vi "PeriodicTaskChannels.vi"(7 "Error In":errorcluster, 8 "Display Type":enum8{"Matrix", "7 Segment"}(ring), 9 "Channels":T1, 10 "LINX Resource":T2) -> (0 "Error Out":errorcluster, 2 "Response":u8[](array[numeric]), 3 "LINX Resource":T2)   [LabVIEW 2019, in "LMH-LINX.lvlib" / "Interaction Parts Kit.lvlib"]
doc: "Updates the Channels used in the Periodic Task using a Custom Command"
uses:
  <vilib>/MakerHub/LINX/Public/Sensors/Digilent/Interaction Parts Kit/Interaction Parts Kit.lvlib
  <vilib>/MakerHub/LINX/Private/Type Defs/LINX Ref.ctl
  <vilib>/MakerHub/LINX/Private/Type Defs/Platform.ctl
  <vilib>/MakerHub/LINX/Private/Type Defs/Interface.ctl
  <vilib>/MakerHub/LINX/Private/Device/Type Defs/LINX Device Config.ctl
  <vilib>/MakerHub/LINX/Private/Device/Type Defs/TCP Config.ctl
  <vilib>/MakerHub/LINX/Private/Device/Type Defs/Channels.ctl
  <vilib>/MakerHub/LINX/LMH-LINX.lvlib
  <vilib>/MakerHub/LINX/Private/Device/Device.lvlib
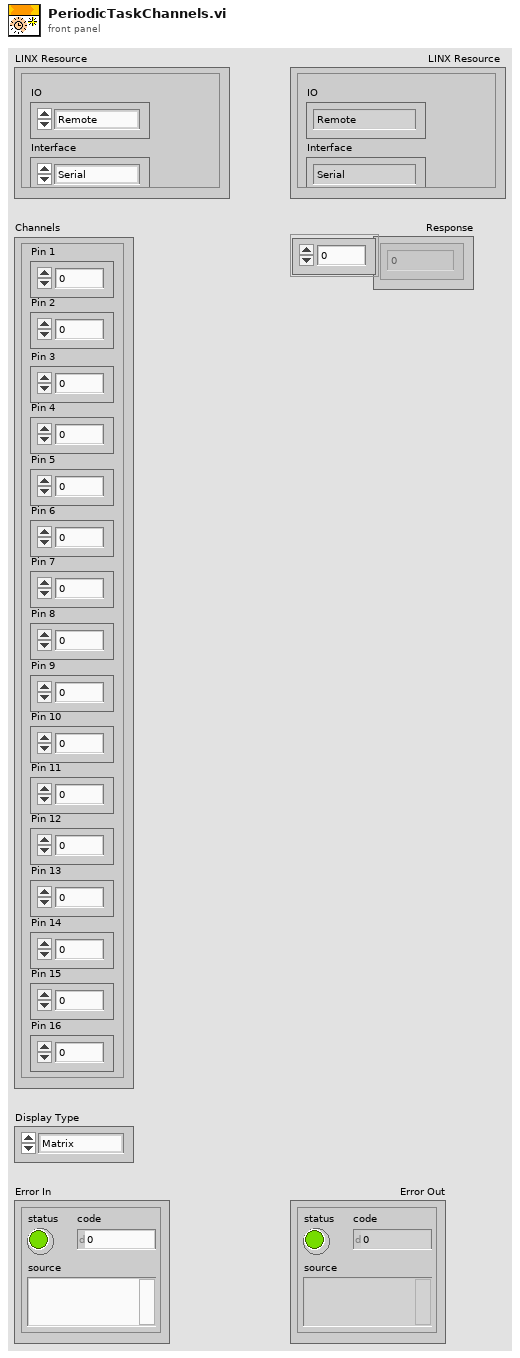
[diagram p1: front panel]
types:
  T1 = cluster{"Pin 1":u8, "Pin 2":u8, "Pin 3":u8, "Pin 4":u8, "Pin 5":u8, "Pin 6":u8, "Pin 7":u8, "Pin 8":u8, "Pin 9":u8, "Pin 10":u8, "Pin 11":u8, "Pin 12":u8, "Pin 13":u8, "Pin 14":u8, "Pin 15":u8, "Pin 16":u8}
  T2 = typedef "LMH-LINX.lvlib/LINX Ref.ctl" = cluster{"IO":T3, "Interface":T4, "LINX Device Config":T5}
  T3 = typedef "LMH-LINX.lvlib/Platform.ctl" = enum16{"Remote", "Local"}
  T4 = typedef "LMH-LINX.lvlib/Interface.ctl" = enum16{"Serial", "TCP"}
  T5 = typedef "LMH-LINX.lvlib/Device.lvlib/LINX Device Config.ctl" = cluster{"Interface":T4, "COM Port":refnum<visa-resource-name>, "TCP Configuration":T6, "Device Family":u8, "Device ID":u8, "Device Name":string, "TCP Ref":refnum<k5>, "Channels":T7}
  T6 = typedef "LMH-LINX.lvlib/Device.lvlib/TCP Config.ctl" = cluster{"IP Address":string, "Port":u16}
  T7 = typedef "LMH-LINX.lvlib/Channels.ctl" = cluster{"DI":u8[], "DO":u8[], "AI":u8[], "AO":u8[], "PWM":u8[], "QE":u8[], "UART":u8[], "I2C 2":u8[], "SPI":u8[], "CAN":u8[], "Servo":u8[], "AI Ref (V)":dbl, "AI Resolution (Bits)":u8, "AO Ref (V)":dbl, "AO Resolution (Bits)":u8}
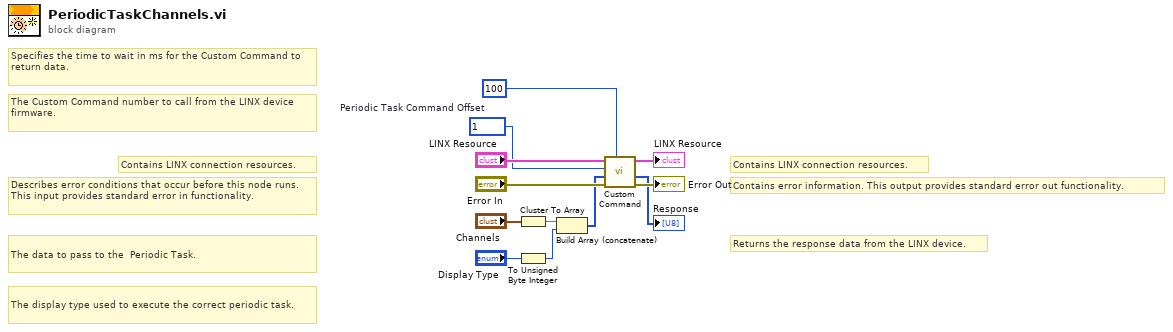
[diagram p0: block diagram]
diagram:
  w10 = u16 1  # Periodic Task Command Offset
  # "The display type used to execute the correct periodic task."
  # "The data to pass to the  Periodic Task."
  # "Specifies the time to wait in ms for the Custom Command to return data."
  # "The Custom Command number to call from the LINX device firmware."
  # "Returns the response data from the LINX device."
  # "Contains LINX connection resources."
  # "Contains error information. This output provides standard error out functionality."
  # "Contains LINX connection resources."
  # "Describes error conditions that occur before this node runs. This input provides standard error in functionality."
  n1 = Cluster To Array(cluster="Channels") -> (array=w1:u8[])
  n2 = To Unsigned Byte Integer(number="Display Type") -> (unsigned 8bit integer=w3:u8)
  n3 = Build Array (concatenate)(w1, w3) -> (w5:u8[])
  n4 = call <vilib>:"Custom Command.vi"("Timeout (100 ms)"=100, "Error In"="Error In", "Data"=w5, "Custom Command Number"=w10, "LINX Resource"="LINX Resource") -> ("Error Out"=→"Error Out":errorcluster, "Response"=→"Response":u8[], "LINX Resource"=→"LINX Resource":T2)  [unwired: 3 in, 1 out]
